vi "Get Windows Path.vi"(8 "error in (no error)":errorcluster) -> (0 "error out":errorcluster, 3 "windows directory":path)   [LabVIEW 2023, in "Winsys.lvlib"]
doc: "Gets the path to the Windows directory."
uses:
  Winsys.lvlib
  WINUTIL/WINUTIL.lvlib
  kernel32.dll
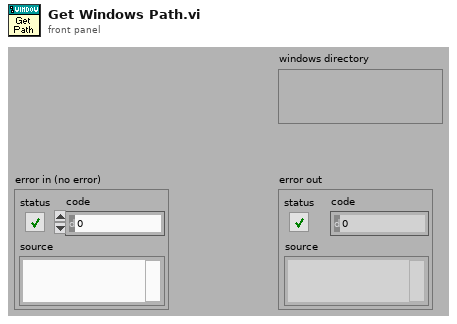
[diagram p1: front panel]
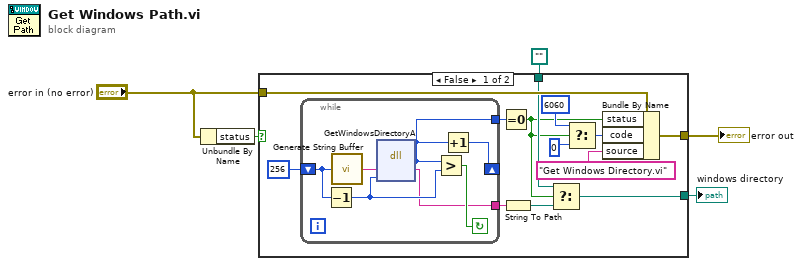
[diagram p0: block diagram]
diagram:
  n1 = Unbundle By Name("error in (no error)") -> ("status"=w5:bool)
  n2 = case shown="False" w5 {
    tunnel: "error in (no error)" -> [w16 w26]
    tunnel: path "" -> [w10 w27]
    tunnel: [w7 w27] -> w3
    tunnel: [w6 w26] -> w1
    frame False {
      n3 = while {
        tunnel: [w19] -> w17
        tunnel: [w20] -> w11
        shift-left: 256 -> [w24]
        shift-right: [w21] -> _
        stop <- w22 continue-if-true
        n4 = Decrement(x=w24) -> (x-1=w23:i32)
        n5 = call "Generate String Buffer.vi"("buffer size"=w24) -> ("string buffer"=w25:string)
        n6 = dll-call lib="kernel32.dll" fn="GetWindowsDirectoryA"("szDir"=w25, "len"=w23) -> (w19:i32, "szDir"=w20:string)  [unwired: 4 in, 2 out]
        n7 = Greater?(x=w19, y=w23) -> (0:w22:bool)
        n8 = Increment(x=w19) -> (x+1=w21:i32)
      }
      n9 = Equal To 0?(x=w17) -> (x = 0?=w9:bool)
      n10 = String To Path(string=w11) -> (path=w8:path)
      n11 = Select(t=w10, s=w9, f=w8) -> (s? t:f=w7:path)
      n12 = Select(t=6060, s=w9, f=0) -> (s? t:f=w15:i32)
      n13 = Bundle By Name(cluster=w16, "status"=w9, "code"=w15, "source"="Get Windows Directory.vi") -> (w6:errorcluster)
    }
    frame True {
    }
  }
  "windows directory" <- w3
  "error out" <- w1
